vi "Read Version.vi"(8 "error in (no error)":errorcluster, 11 "KObject in":refnum<class "KObject.lvclass">) -> (0 "error out":errorcluster, 2 "Version":i32, 3 "KObject out":refnum<class "KObject.lvclass">)   [LabVIEW 2020, in "KObject.lvclass"]
uses:
  KObject.lvclass
  KObject.lvclass/KObject.ctl
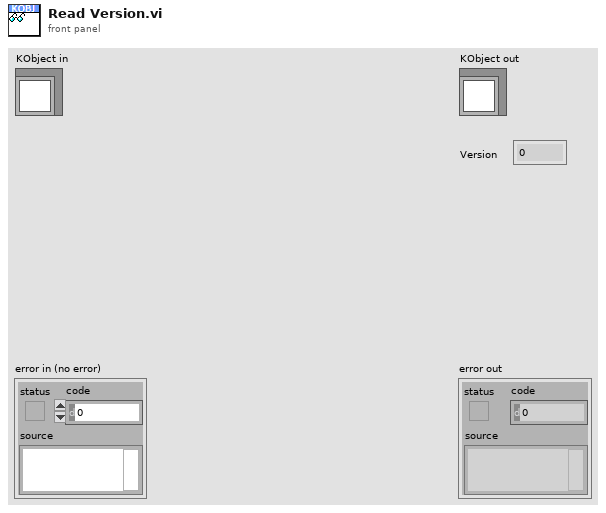
[diagram p1: front panel]
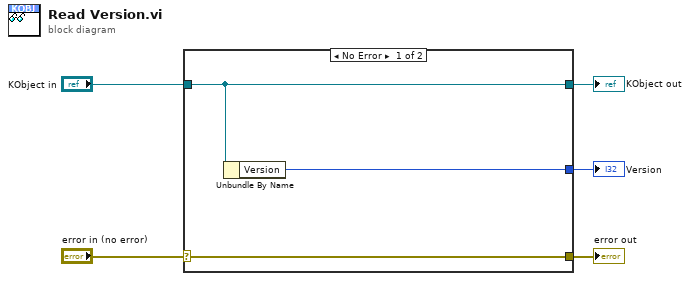
[diagram p0: block diagram]
diagram:
  n1 = case shown="No Error" "error in (no error)" {
    selector: "error in (no error)" -> [w8 w9]
    tunnel: [w8 w9] -> w4
    tunnel: [w7 w10] -> w2
    tunnel: "KObject in" -> [w7 w10]
    tunnel: [w6 _] -> w1
    frame No Error {
      n2 = Unbundle By Name(w7) -> ("Version"=w6:i32)
    }
    frame Error {
    }
  }
  "error out" <- w4
  "KObject out" <- w2
  "Version" <- w1
